vi "Get XLXS Cell Span Information.vi"(8 "Error In":errorcluster, 11 "String":string) -> (0 "Error Out":errorcluster, 2 "Cell Span":T1(array[cluster]), 3 "String dup":string)   [LabVIEW 2021, in "Files.lvlib"]
doc: "Reads the section of the file containing information on cells spanning multiple elementary cells and returns an array of clusters containing the top-left and bottom-right coordinates of each cell."
uses:
  Files.lvlib
panel:
  # "see the AlliGator License on the block diagram (Ctrl+E or Window:Show Block Diagram)"
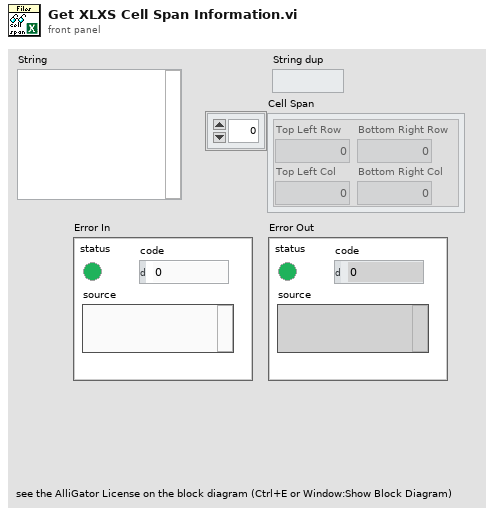
[diagram p1: front panel]
types:
  T1 = cluster{"Top Left Row":i32, "Top Left Col":i32, "Bottom Right Row":i32, "Bottom Right Col":i32}[]
  T2 = cluster{"Top Left Row":i32, "Top Left Col":i32, "Bottom Right Row":i32, "Bottom Right Col":i32}
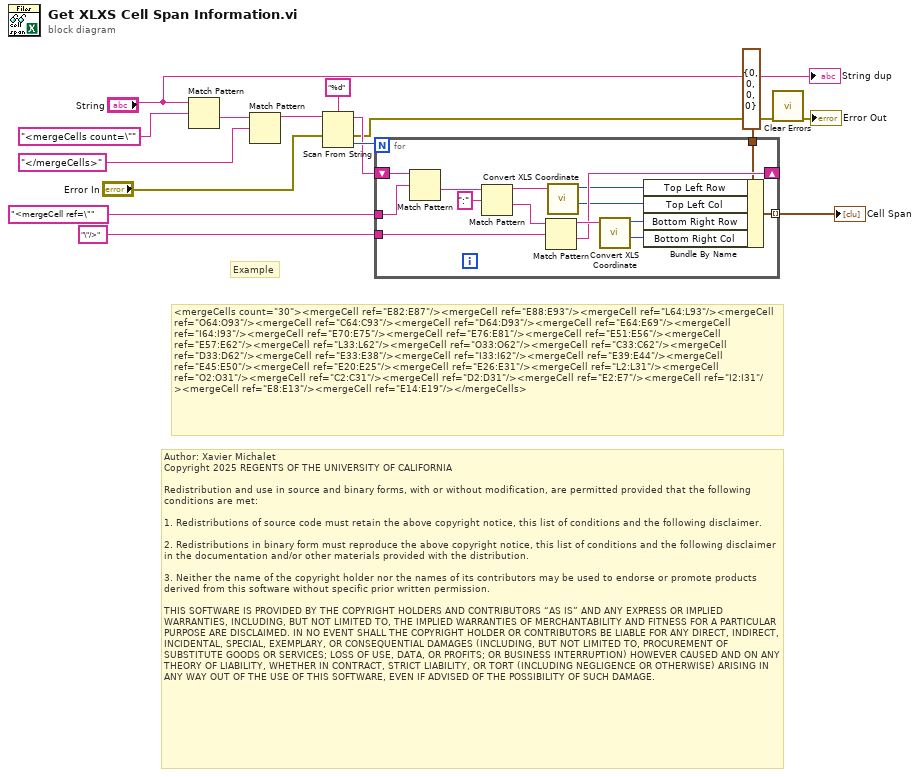
[diagram p0: block diagram]
diagram:
  # "Example"
  # "Author: Xavier Michalet\nCopyright 2025 REGENTS OF THE UNIVERSITY OF CALIFORNIA\n\nRedistribution and use in source and binary forms, with or without modification, are permitted provided that the following conditions are met:\n\n1. Redistributions of source code must retain the above copyright notice, this list of conditions and the following disclaimer.\n\n2. Redistributions in binary form must reproduce the above copyright notice, this list of conditions and the following disclaimer in the documentation and/or other materials provided with the distribution.\n\n3. Neither the name of the copyright holder nor the names of its contributors may be used to endorse or promote products derived from this software without specific prior written permission.\n\nTHIS SOFTWARE IS PROVIDED BY THE COPYRIGHT HOLDERS AND CONTRIBUTORS “AS IS” AND ANY EXPRESS OR IMPLIED WARRANTIES, INCLUDING, BUT NOT LIMITED TO, THE IMPLIED WARRANTIES OF MERCHANTABILITY AND FITNESS FOR A PARTICULAR PURPOSE ARE DISCLAIMED. IN NO EVENT SHALL THE COPYRIGHT HOLDER OR CONTRIBUTORS BE LIABLE FOR ANY DIRECT, INDIRECT, INCIDENTAL, SPECIAL, EXEMPLARY, OR CONSEQUENTIAL DAMAGES (INCLUDING, BUT NOT LIMITED TO, PROCUREMENT OF SUBSTITUTE GOODS OR SERVICES; LOSS OF USE, DATA, OR PROFITS; OR BUSINESS INTERRUPTION) HOWEVER CAUSED AND ON ANY THEORY OF LIABILITY, WHETHER IN CONTRACT, STRICT LIABILITY, OR TORT (INCLUDING NEGLIGENCE OR OTHERWISE) ARISING IN ANY WAY OUT OF THE USE OF THIS SOFTWARE, EVEN IF ADVISED OF THE POSSIBILITY OF SUCH DAMAGE."
  # "<mergeCells count=\"30\"><mergeCell ref=\"E82:E87\"/><mergeCell ref=\"E88:E93\"/><mergeCell ref=\"L64:L93\"/><mergeCell ref=\"O64:O93\"/><mergeCell ref=\"C64:C93\"/><mergeCell ref=\"D64:D93\"/><mergeCell ref=\"E64:E69\"/><mergeCell ref=\"I64:I93\"/><mergeCell ref=\"E70:E75\"/><mergeCell ref=\"E76:E81\"/><mergeCell ref=\"E51:E56\"/><mergeCell ref=\"E57:E62\"/><mergeCell ref=\"L33:L62\"/><mergeCell ref=\"O33:O62\"/><mergeCell ref=\"C33:C62\"/><mergeCell ref=\"D33:D62\"/><mergeCell ref=\"E33:E38\"/><mergeCell ref=\"I33:I62\"/><mergeCell ref=\"E39:E44\"/><mergeCell ref=\"E45:E50\"/><mergeCell ref=\"E20:E25\"/><mergeCell ref=\"E26:E31\"/><mergeCell ref=\"L2:L31\"/><mergeCell ref=\"O2:O31\"/><mergeCell ref=\"C2:C31\"/><mergeCell ref=\"D2:D31\"/><mergeCell ref=\"E2:E7\"/><mergeCell ref=\"I2:I31\"/><mergeCell ref=\"E8:E13\"/><mergeCell ref=\"E14:E19\"/></mergeCells>"
  n1 = Match Pattern(string="String", regular expression="<mergeCells count=\"") -> (after substring=w14:string)  [unwired: 1 in, 3 out]
  n2 = Match Pattern(string=w14, regular expression="</mergeCells>") -> (before substring=w12:string)  [unwired: 1 in, 3 out]
  n3 = Scan From String(format string="%d", input string=w12, error in="Error In") -> (remaining string=w8:string, error out=w3:errorcluster, output 1=w9:i32)  [unwired: 2 in, 1 out]
  n4 = for {
    N: w9 -> [_]
    shift-right: [w22] -> _
    shift-left: w8 -> [w30]
    tunnel: "<mergeCell ref=\"" ("regular expression") -> [w29]
    tunnel: "\"/>" ("regular expression") -> [w24]
    tunnel: [w17] -> w5 mode=indexing
    tunnel: T2 {"Top Left Row"=0, "Top Left Col"=0, "Bottom Right Row"=0, "Bottom Right Col"=0} ("Cell Span") -> [w16]
    n5 = Match Pattern(string=w30, regular expression=w29) -> (after substring=w28:string)  [unwired: 1 in, 3 out]
    n6 = Match Pattern(string=w28, regular expression=":") -> (before substring=w26:string, after substring=w25:string)  [unwired: 1 in, 2 out]
    n7 = Match Pattern(string=w25, regular expression=w24) -> (before substring=w23:string, after substring=w22:string)  [unwired: 1 in, 2 out]
    n8 = call "Convert XLS Coordinate.vi"("Excel coordinate"=w26) -> ("Column"=w20:i32, "Row"=w21:i32)  [unwired: 9 in]
    n9 = call "Convert XLS Coordinate.vi"("Excel coordinate"=w23) -> ("Column"=w18:i32, "Row"=w19:i32)  [unwired: 9 in]
    n10 = Bundle By Name(cluster=w16, "Top Left Row"=w21, "Top Left Col"=w20, "Bottom Right Row"=w19, "Bottom Right Col"=w18) -> (w17:T2)
  }
  "Cell Span" <- w5
  n11 = call <vilib>:"Clear Errors.vi"("error in (no error)"=w3) -> ("error out"=→"Error Out":errorcluster)  [unwired: 5 in, 1 out]
  "String dup" <- "String"
